vi "Create Group Buffers.vi"(8 "error in (no error)":errorcluster, 10 "Framework Configuration":refnum<class "Framework Configuration.lvclass">, 11 "Framework in":refnum<class "Framework.lvclass">) -> (0 "error out":errorcluster, 2 "Group Buffers":refnum<class "Buffers.lvclass">[](array[class]), 3 "Framework out":refnum<class "Framework.lvclass">)   [LabVIEW 2017, in "DSF Core.lvlib" / "Framework.lvclass"]
uses:
  Framework.lvclass
  Buffers/Buffers.lvclass
  Configuration/Core/Framework/Framework Configuration.lvclass
  Configuration/Core/Framework/Framework Configuration.lvclass/Framework Configuration.ctl
  Configuration/Core/Plugin/Plugin Configuration.lvclass/Plugin Configuration.ctl
  Configuration/Core/Thread/Thread Configuration.lvclass/Thread Configuration.ctl
  Buffer/Buffer.lvclass
  C:/Program Files (x86)/National Instruments/LabVIEW 2017/vi.lib/NI/Memory Manager/Classes/Pointer/Pointer.lvclass
  <vilib>/NI/Memory Manager/Classes/Pointer/Pointer.lvclass/Pointer.ctl
  <vilib>/NI/Memory Manager/Classes/Pointer/Set Size.vi
  <vilib>/NI/Memory Manager/Classes/Pointer/Set Address.vi
  <vilib>/NI/Memory Manager/Classes/Pointer/Check Null Pointer.vi
  <vilib>/NI/Memory Manager/Classes/Pointer/Set Internal.vi
  <vilib>/NI/Memory Manager/Classes/Pointer/Errors.vi
  <vilib>/NI/Memory Manager/Classes/Pointer/Null Pointer.vi
  <vilib>/NI/Memory Manager/Classes/Pointer/Is Null.vi
  <vilib>/NI/Memory Manager/Classes/Pointer/Create Error.vi
  <vilib>/NI/Memory Manager/Classes/Pointer/Get Address.vi
  <vilib>/NI/Memory Manager/Constants/Constants.vi
  <vilib>/NI/Memory Manager/Constants/Library Name.vi
  <vilib>/NI/Memory Manager/Classes/Pointer/Pointer Error Info.vi
  <vilib>/NI/Memory Manager/Constants/Pointer Class Name.vi
  <vilib>/NI/Memory Manager/VIs/New Error Cluster.vi
  <vilib>/NI/Memory Manager/VIs/New Error Cluster (512B).vi
  <vilib>/NI/Memory Manager/VIs/Set Error Status.vi
  <vilib>/NI/Memory Manager/VIs/Set Error Code.vi
  <vilib>/NI/Memory Manager/VIs/Set Error Source.vi
  <vilib>/NI/Memory Manager/VIs/Write String to Source.vi
  Configuration/Core/Group/Group Configuration.lvclass
  Configuration/Core/Plugin/Plugin Configuration.lvclass
  <vilib>/NI/Memory Manager/Classes/Pointer/Pointer.lvclass
  Configuration/Core/Thread/Thread Configuration.lvclass
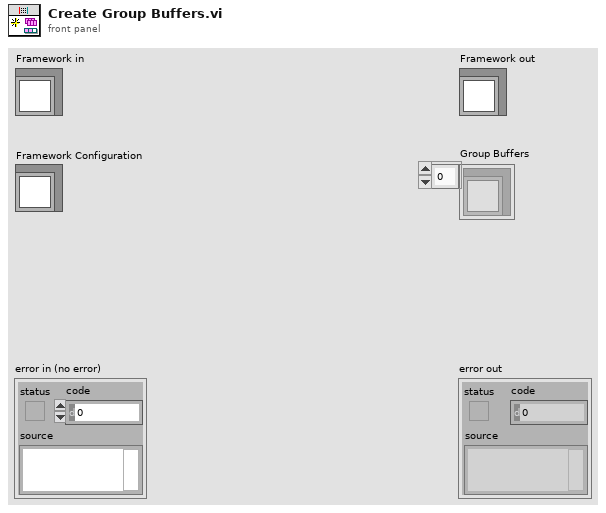
[diagram p1: front panel]
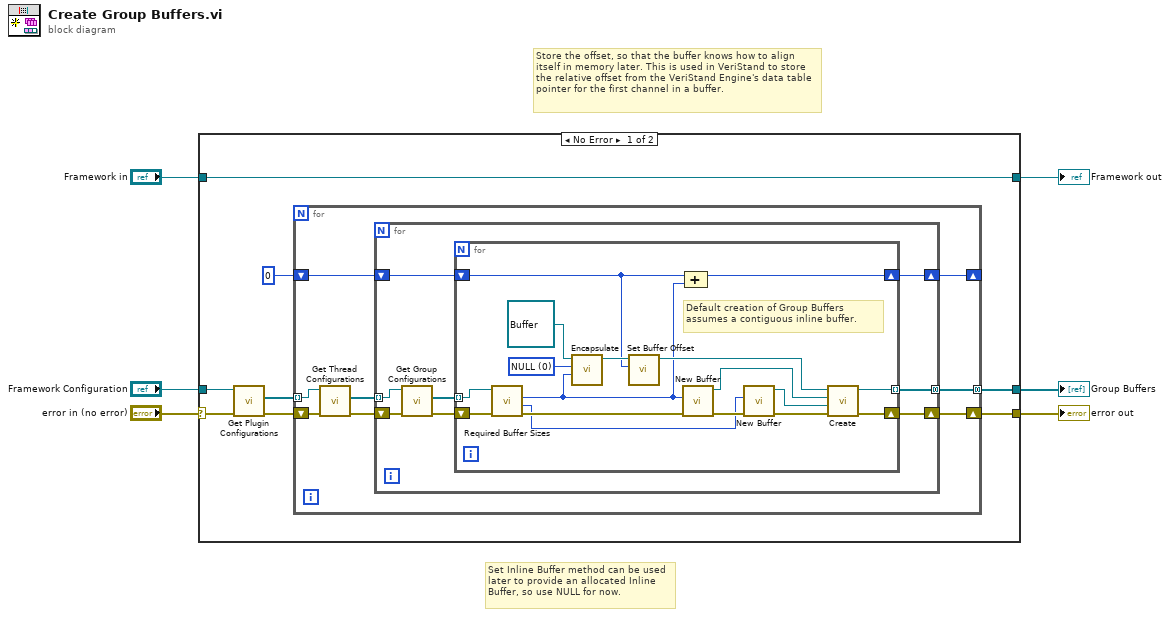
[diagram p0: block diagram]
diagram:
  # "Store the offset, so that the buffer knows how to align itself in memory later. This is used in VeriStand to store the relative offset from the VeriStand Engine's data table pointer for the first channel in a buffer."
  # "Set Inline Buffer method can be used later to provide an allocated Inline Buffer, so use NULL for now."
  n1 = case shown="No Error" "error in (no error)" {
    selector: "error in (no error)" -> [w10 w49]
    tunnel: [w9 w49] -> w5
    tunnel: [w14 w48] -> w3
    tunnel: "Framework in" -> [w14 w48]
    tunnel: "Framework Configuration" -> [w11 _]
    tunnel: [w8 _] -> w1
    frame No Error {
      n2 = call "Get Plugin Configurations.vi"("error in (no error)"=w10, "Framework Configuration in"=w11) -> ("error out"=w12:errorcluster, "Plugin Configurations"=w13:refnum<class "Plugin Configuration.lvclass">[])  [unwired: 7 in, 1 out]
      n3 = for {
        tunnel: w13 -> [w22] mode=indexing
        shift-right: [w18] -> w9
        shift-left: w12 -> [w20]
        tunnel: [w17] -> w8 mode=concatenating
        shift-right: [w15] -> _
        shift-left: u64 0 ("engine size") -> [w16]
        n4 = call "Get Thread Configurations.vi"("error in (no error)"=w20, "Plugin Configuration in"=w22) -> ("error out"=w19:errorcluster, "Thread Configurations"=w21:refnum<class "Thread Configuration.lvclass">[])  [unwired: 7 in, 1 out]
        n5 = for {
          tunnel: w21 -> [w30] mode=indexing
          shift-right: [w26] -> w18
          shift-left: w19 -> [w28]
          tunnel: [w25] -> w17 mode=concatenating
          shift-right: [w23] -> w15
          shift-left: w16 -> [w24]
          n6 = call "Get Group Configurations.vi"("error in (no error)"=w28, "Thread Configuration in"=w30) -> ("error out"=w27:errorcluster, "Group Configurations"=w29:refnum<class "Group Configuration.lvclass">[])  [unwired: 7 in, 1 out]
          n7 = for {
            tunnel: w29 -> [w34] mode=indexing
            shift-right: [w41] -> w26
            shift-left: w27 -> [w33]
            tunnel: [w40] -> w25 mode=indexing
            shift-right: [w39] -> w23
            shift-left: w24 -> [w35]
            w45 = u64 0 items=["NULL"] ("Null")
            # "Default creation of Group Buffers assumes a contiguous inline buffer."
            n8 = call-dynamic "Required Buffer Sizes.vi"("error in (no error)"=w33, "Group Configuration in"=w34) -> ("error out"=w32:errorcluster, "string size"=w31:u64, "engine size"=w36:u64)  [unwired: 6 in, 1 out]
            n9 = call <vilib>:"Encapsulate.vi"("size"=w36, "address"=w45, "Pointer type"=refnum<class "Buffer.lvclass"> refnum ("Inline Buffer (null)")) -> ("Pointer"=w38:refnum<class "Buffer.lvclass">)  [unwired: 7 in, 1 out]
            n10 = call "Set Buffer Offset.vi"("buffer offset"=w35, "Buffer in"=w38) -> ("Buffer out"=w37:refnum<class "Buffer.lvclass">)  [unwired: 9 in]
            n11 = call "New Buffer.vi"("error in (no error)"=w32, "buffer size"=w36) -> ("error out"=w47:errorcluster, "Buffer out"=w43:refnum<class "Buffer.lvclass">)  [unwired: 8 in]
            n12 = Compound Arithmetic op=ADD(w35, w36) -> (w39:u64)
            n13 = call "New Buffer.vi"("error in (no error)"=w47, "buffer size"=w31) -> ("error out"=w42:errorcluster, "Buffer out"=w46:refnum<class "Buffer.lvclass">)  [unwired: 8 in]
            n14 = call "Create.vi"("error in (no error)"=w42, "String Buffer (null)"=w46, "Async Buffer (null)"=w43, "Inline Buffer (null)"=w37) -> ("error out"=w41:errorcluster, "Buffers out"=w40:refnum<class "Buffers.lvclass">)  [unwired: 6 in]
          }
        }
      }
    }
    frame Error {
    }
  }
  "error out" <- w5
  "Framework out" <- w3
  "Group Buffers" <- w1
